vi "ConcatenateNonBlanks.vi"(1 "separator":string=";", 5 "prependString":string, 9 "appendString":string, 12 "uniqueOnly":bool) -> (8 "outputString":string)   [LabVIEW 2020]
doc: "Concatenates strings, WITHOUT putting separators where the string are null or whitespace"
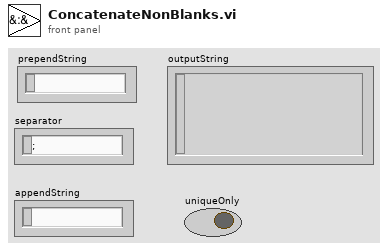
[diagram p1: front panel]
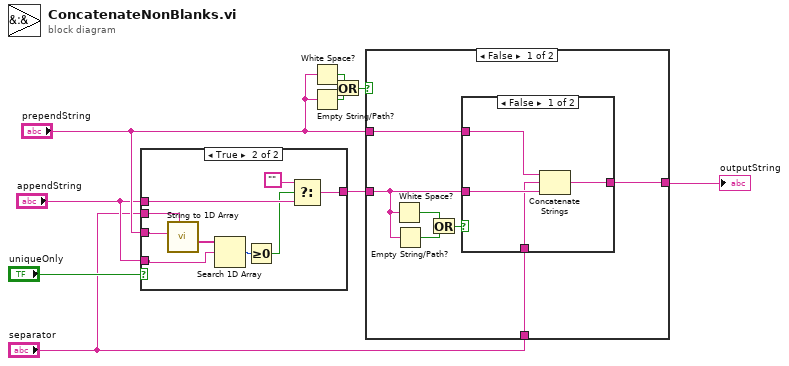
[diagram p0: block diagram]
diagram:
  n1 = case shown="True" "uniqueOnly" {
    tunnel: "prependString" -> [_ w16]
    tunnel: "appendString" -> [_ w14]
    tunnel: "appendString" -> [w10 w18]
    tunnel: [w10 w19] -> w2
    tunnel: "separator" -> [_ w11]
    frame False {
    }
    frame True {
      n2 = call "String to 1D Array.vi"("delimiter (Tab)"=w11, "string"=w16) -> ("Array of Strings"=w15:string[])  [unwired: 9 in]
      n3 = Search 1D Array(1D array=w15, element=w14) -> (index of element=w13:i32)  [unwired: 1 in]
      n4 = Greater Or Equal To 0?(x=w13) -> (x >= 0?=w12:bool)
      n5 = Select(t="", s=w12, f=w18) -> (s? t:f=w19:string)
    }
  }
  n6 = White Space?(1:"prependString") -> (0:w8:bool)
  n7 = Empty String/Path?(string/path="prependString") -> (empty?=w6:bool)
  n8 = Or(x=w8, y=w6) -> (x .or. y?=w7:bool)
  n9 = case shown="False" w7 {
    tunnel: w2 -> [w22 w32]
    tunnel: [w26 w32] -> w9
    tunnel: "prependString" -> [w25 _]
    tunnel: "separator" -> [w24 _]
    frame False {
      n10 = White Space?(1:w22) -> (0:w21:bool)
      n11 = Empty String/Path?(string/path=w22) -> (empty?=w23:bool)
      n12 = Or(x=w21, y=w23) -> (x .or. y?=w20:bool)
      n13 = case shown="False" w20 {
        tunnel: w22 -> [w30 _]
        tunnel: [w29 w31] -> w26
        tunnel: w25 -> [w28 w31]
        tunnel: w24 -> [w27 _]
        frame False {
          n14 = Concatenate Strings(w28, w27, w30) -> (w29:string)
        }
        frame True {
        }
      }
    }
    frame True {
    }
  }
  "outputString" <- w9
